vi "Print Features Report.vi"(6 "Local Data in":T2, 7 "UI References":T1, 8 "error in (no error)":errorcluster) -> (0 "error out":errorcluster)   [LabVIEW 2024]
uses:
  Controls/Print Command.ctl
  Controls/Language Vision Text Cluster.ctl
  Controls/RVHR - Reporting Settings.ctl
  Controls/RVHR - Local Data.ctl
  Controls/Test Cluster.ctl
  Controls/Excluded Information.ctl
  Controls/Language.ctl
  Controls/Device_Type.ctl
  <vilib>/Utility/miscctls.llb/LVRectTypeDef.ctl
  <vilib>/Utility/miscctls.llb/LVBoundsTypeDef.ctl
  Controls/RVHR - UI Refs.ctl
  <vilib>/drjdpowell/SQLite Library/SQL Connection/Open (path).vi
  <vilib>/drjdpowell/SQLite Library/SQL Connection/Open (string).vi
  <vilib>/AdvancedString/Path To Command Line String.vi
  <vilib>/drjdpowell/SQLite Library/SQL Connection/Execute SQL.vi
  <vilib>/drjdpowell/SQLite Library/SQL Connection/Connection.lvclass
  <vilib>/Exaprom PDF/Controls/Image Controls/Image aligment.ctl
  <vilib>/Exaprom PDF/Controls/Image Controls/Image alignment and position.ctl
  <vilib>/Exaprom PDF/Controls/Image Controls/Image border.ctl
  <vilib>/Exaprom PDF/Controls/Initialization Controls/At the opening.ctl
  <vilib>/Exaprom PDF/Controls/Page Controls/Page margins.ctl
  <vilib>/Exaprom PDF/Controls/Page Controls/Page Layout Custom.ctl
  <vilib>/Exaprom PDF/Controls/Page Controls/Page Orientation.ctl
  <vilib>/Exaprom PDF/Controls/Page Controls/Page size.ctl
  <vilib>/Exaprom PDF/Controls/Page Controls/Page setup.ctl
  <vilib>/Exaprom PDF/Controls/Initialization Controls/PDF Details.ctl
  <vilib>/Exaprom PDF/Controls/Text Controls/Unicode/Type and run direction.ctl
  <vilib>/Exaprom PDF/Controls/Font Controls/Type and encoding.ctl
  <vilib>/Exaprom PDF/Controls/Font Controls/Font color.ctl
  <vilib>/Exaprom PDF/Controls/Font Controls/Font size.ctl
  <vilib>/Exaprom PDF/Controls/Font Controls/Font complete cluster.ctl
  <vilib>/Exaprom PDF/Controls/Initialization Controls/Image or Table Caption.ctl
  <vilib>/Exaprom PDF/Controls/Initialization Controls/Captions.ctl
  <vilib>/Exaprom PDF/Controls/Text Controls/Line spacing.ctl
  <vilib>/Exaprom PDF/Controls/Text Controls/Texte alignement.ctl
  <vilib>/Exaprom PDF/Controls/Initialization Controls/Defaut Paragraphe and Line Spacing.ctl
  <vilib>/Exaprom PDF/Controls/Initialization Controls/File Permission Parameters.ctl
  <vilib>/drjdpowell/SQLite Library/SQLite.lvlib
panel:
  out "Column Names 2":string[](array[string])
  out "Feature Table":string[][](array[string])
  out "Local Data out":T2
  in  "Settings":T9
  in  "Language Config Cluster":T10={"Home"="Home", "Test Setup"="Setup", "Run Test"="Test", "Configure"="Config", "Hardware Viewer"="Viewer", "Review Test"="Review", "Report"="Home", "Exit"="Exit", "Device Connected?"="Device Connected?", "Test in Progress?"="Test in Progress?", "Simulate?"="Simulate?", "Device Type 1"="Corrugation Analysis Trolley", "Device Type 2"="Bi-Corrugation Analysis Trolley", "Device Type 3"="Bi-Corrugation Analysis Trolley", "Device Type 4"="Bi-Corrugation Analysis Trolley", "Device Type 5"="Bi-Corrugation Analysis Trolley", "Device Type 6"="Bi-Corrugation Analysis Trolley", "Device Type 7"="Bi-Corrugation Analysis Trolley", "Software Version"="Version", "Support"="Software by RailMeasurement Limited - Cambridge - UK - support@railmeasurement.com", "Operator"="Operator:", "Test Description"="Description:", "Line"="Description:", "Test Folder Path"="Folder Path:", "Test Folder Path RCA"="Folder Path:", "Start Position"="Start Position:", "Sensor Position"="Sensor Position:", "Sensor A Position"="Sensor A Position:", "Sensor B Position"="Sensor B Position:", "Visible Chart Distance"="Sensor B Position:", "Rail Side"="Rail Side:", "Rail A Side"="Rail A Side:", "Distance Direction"="Distance Direction:", "Start"="Start:", "Distance Travelled"="Distance Travelled:", "Current Position"="Current Position:", "Stop Test"="Stop", "Pause Test"="Save", "Displacement"="Displacement", "Position"="Position", "Sensor Calibration"="Sensor Calibration:", "Sensor A Calibration"="Sensor A Calibration:", "Sensor B Calibration"="Sensor B Calibration:", "Encoder Spacing"="Encoder Spacing:", "Sampling Distance"="Sampling Distance:", "Tacho Pulses/Rev"="Sensor Calibration:", "Wheel Diameter"="Sensor A Calibration:", "Sampling Distances"=["1mm", "2mm"], "Distance Unit"="Distance in:", "Distance Units"=["Kilometres", "miles & chains", "metres", "stations", "miles"], "Swap Direction"="Swap Direction at Run End?", "Language"="Language", "Device Resolution"="Save", "Device Resolutions"=["Kilometres", "miles & chains", "metres", "stations", "miles"], "Detect Change in Direction"="Save", "Save Config"="Save", "Encoder Data"="Encoder Data", "Sensor Data"="Sensor Data", "Sensor A Data"="Sensor A Data", "Sensor B Data"="Sensor B Data", "Voltage"="Voltage", "Time (m:s)"="Time (m:s)", "Unit mm/s/V"="(mm/s)/V", "Unit mm"="mm", "Unit km"="km", "Unit m"="m", "Start Test Message"="m", "Stop Test Message"="km", "Exit Message"="mm", "File Exists Message"="mm", "File Path Invalid Message"="mm", "Combine Error"="mm", "Combine Success"="mm", "Roller Comp Error"="mm", "Test Folder Path (Live)"="mm", "Folder Error"="Sensor B Position:", "Enc Count"="Setup", "Run Start"="mm", "Run End"="mm", "Date"="mm", "Train"="Sensor B Position:", "Location"="Setup", "Notes"="mm", "Heading_1"="mm", "Heading_2"="mm", "Left Rail"="Sensor B Position:", "Right Rail"="Setup", "Left Exclusions"="mm", "Right Exclusions"="mm", "Settings"="mm", "Wavelength Ranges"="Sensor B Position:", "Y-Axis Limits"="Setup", "Exc Limits"="Sensor B Position:", "Other Settings"="Setup", "Distance/Page"="mm", "Distance/Pages"=["Kilometres", "miles & chains", "metres", "stations", "miles"], "Gridlines"="mm", "Report Tolerance"="mm", "Manual Cut"="Sensor B Position:", "Plot Colour"="Distance in:", "Plot Colours"=["Kilometres", "miles & chains", "metres", "stations", "miles"], "EN Standard"="mm", "RiL Standard"="mm", "Custom Standard"="mm", "Resolution"="Distance in:", "Resolutions"=["Kilometres", "miles & chains", "metres", "stations", "miles"], "Exceedence Header"="mm", "Distance (km)"="mm", "Left (%)"="mm", "Right (%)"="Distance in:", "Page"="Distance in:", "Align"="mm", "Main"="mm", "Comparison"="Distance in:", "Offset"="Distance in:", "From"="Distance in:", "To"="Distance in:", "Of"="Distance in:", "File"="mm", "Load New"="mm", "Load Comparison"="Distance in:", "Discard Comparison"="Distance in:", "Print Current Page"="Distance in:", "Print All Pages"="Distance in:", "Print Exceedence Report"="Distance in:", "Plot Main"="Distance in:", "No Comparison Data to Align"="Distance in:", "Run Load Error"="Distance in:", "Report Load Error"="Distance in:", "Cut"="Distance in:", "Remove"="Distance in:", "Config Settings Unsaved"="Distance in:", "Acquisition Paused"="Distance in:", "Please Select One Option Below"="Distance in:", "RCA is Now Stationary"="Distance in:", "Reporting Setting"="Distance in:", "Main Abbreviated"="Distance in:", "Comparison Abbreviated"="Distance in:", "Exceedence Abbreviated"="Distance in:", "Align Comparison"="Distance in:", "Rail Corrugation Analyser Reporting"="Distance in:", "Show Exc. % in Graph"="Distance in:", "Evaluate Sections <100m"="Distance in:", "Evaluate Sections <0.062mile"="Distance in:", "Section Too Short for Evaluation"="Distance in:", "Language Change Prompt"="Distance in:", "Show All"="Distance in:", "Sections_km"="Distance in:", "Sections_mi"="Distance in:", "Vision"="Distance in:", "Vision Report"="Distance in:", "Vision Display"="Distance in:", "Vision Displays"=["Kilometres", "miles & chains", "metres", "stations", "miles"], "Save Images"="Distance in:", "Image Frequency"="Distance in:", "Section"="Distance in:", "Brightness"="Distance in:", "Contrast"="Distance in:", "Shadow"="Distance in:", "Sharpened"="Distance in:", "Apply to all Images"="Distance in:", "Reset"="Distance in:", "Are you sure"="Distance in:", "Image Processing"="Distance in:", "Save Video"="Distance in:", "Image Offset"="Distance in:", "Camera Mode"="Distance in:", "Camera Modes"=["Kilometres", "miles & chains", "metres", "stations", "miles"], "Copy Page"="Distance in:", "Copy Graphs"="Distance in:", "Camera Mode Change Prompt"="Distance in:", "Camera_1 Missing"="Distance in:", "Camera_2 Missing"="Distance in:", "Cameras Missing"="Distance in:", "Camera Setup"="Distance in:", "Camera_1 Connection Error"="Distance in:", "Camera_2 Connection Error"="Distance in:", "Cameras Connection Error"="Distance in:", "No GPS"="Distance in:", "No Signal"="Distance in:", "Camera_1 Connected"="Distance in:", "Camera_1 Not Connected"="Distance in:", "Camera_2 Connected"="Distance in:", "Camera_2 Not Connected"="Distance in:", "Start Position at 0m?"="Distance in:", "Continue"="Distance in:", "New Test, Same Direction"="Distance in:", "New Test, Opposite Direction"="Distance in:", "Stop and Save"="Distance in:", "Live Corrug Estimate"="Distance in:", "Wavelength Corrug"="Distance in:", "Distance Corrug "="Distance in:", "Update Corrug"="Distance in:", "Company"="Distance in:", "Ref Profile "="Distance in:", "Company_Report"="Distance in:", "Ref Profile_Report"="Distance in:", "Heading_1_RVHR"="Distance in:", "Heading_2_RVHR"="Distance in:", "Remove Feature"="Distance in:", "Feature Type"="Sampling Distance:", "Feature Types"=["1mm", "2mm"], "AI Not Ready"="Sampling Distance:"}
  in  "Command":T11
  in  "Main VI Path":path
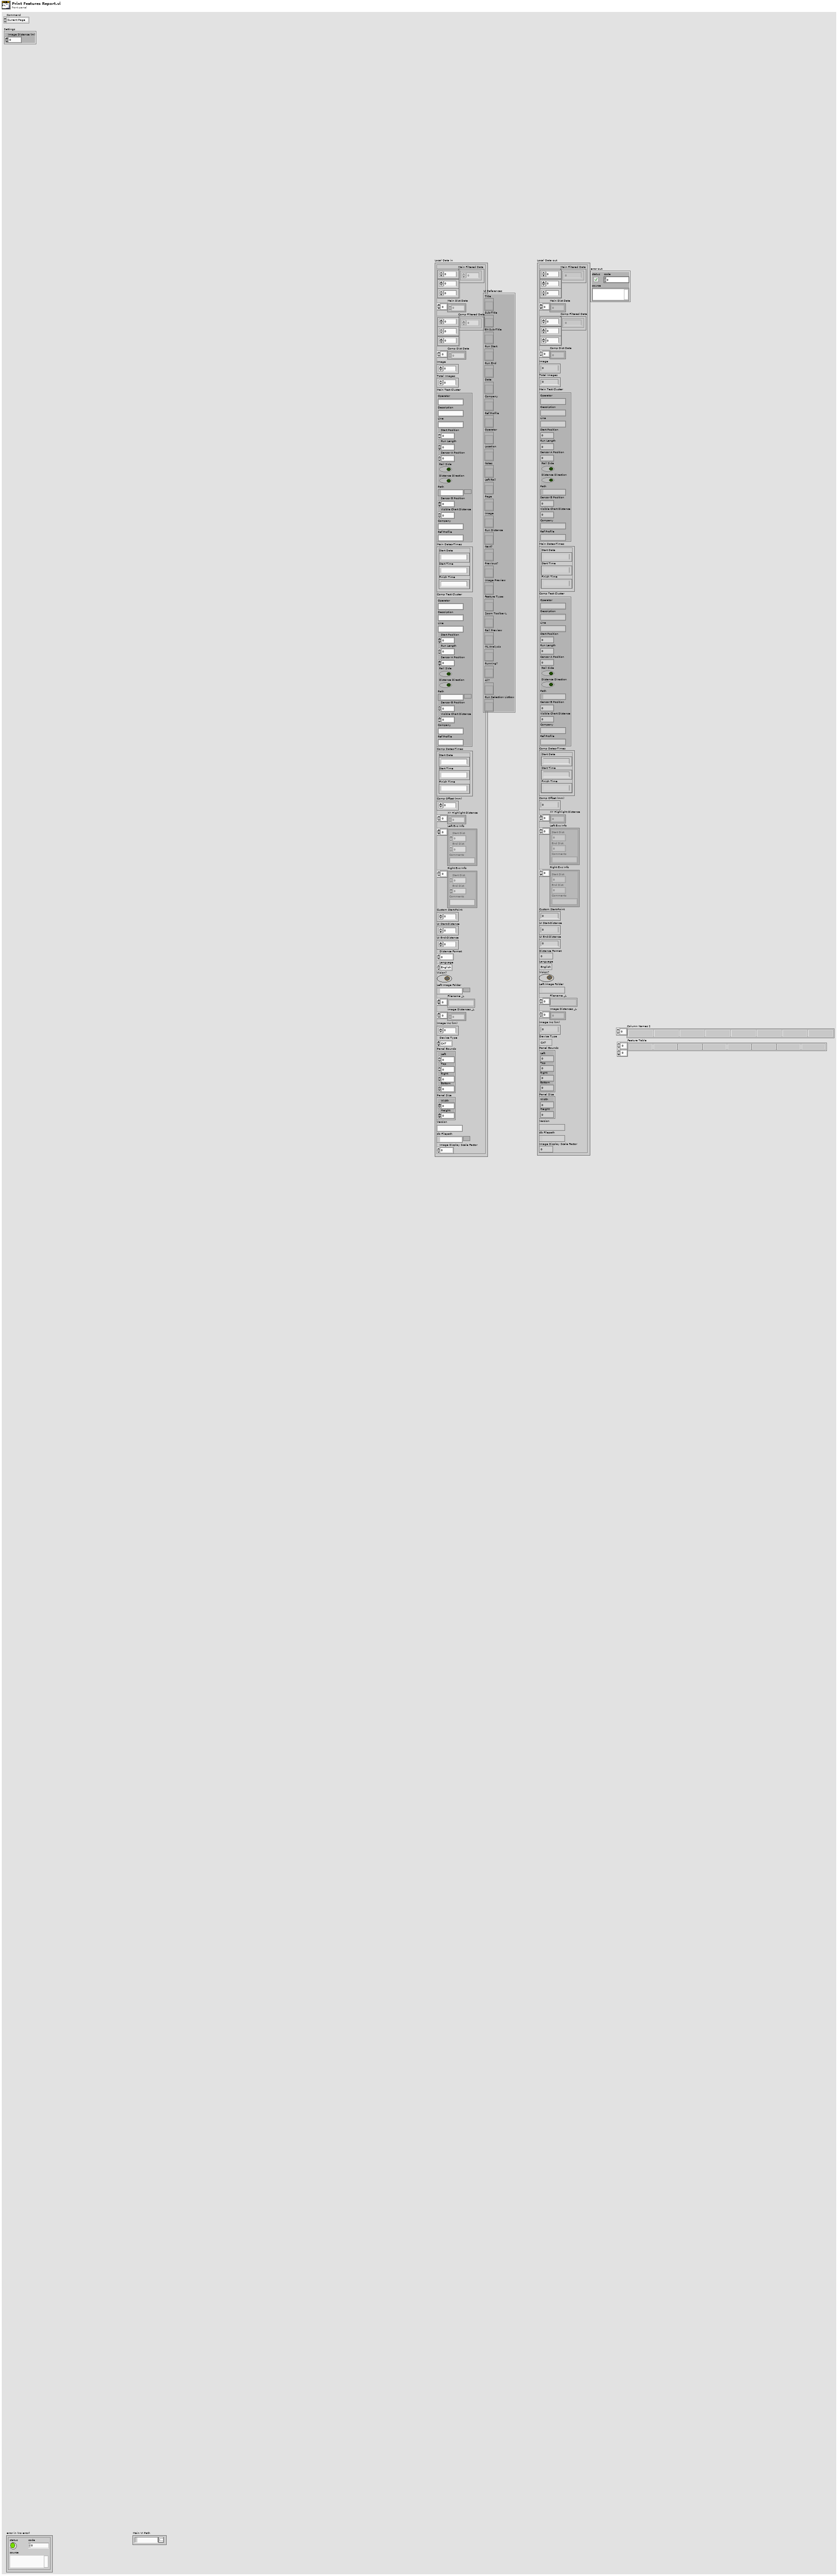
[diagram p1: front panel]
types:
  T1 = typedef "RVHR - UI Refs.ctl" = cluster{"Title":refnum<vi>, "Sub-Title":refnum<vi>, "EN Sub-Title":refnum<vi>, "Run Start":refnum<vi>, "Run End":refnum<vi>, "Date":refnum<vi>, "Company":refnum<vi>, "Ref Profile":refnum<vi>, "Operator":refnum<vi>, "Location":refnum<vi>, "Notes":refnum<vi>, "Left Rail":refnum<vi>, "Page":refnum<vi>, "Image":refnum<vi>, "Run Distance":refnum<vi>, "Next?":refnum<vi>, "Previous?":refnum<vi>, "Image Preview":refnum<vi>, "Feature Type:":refnum<vi>, "Zoom Toolbar L":refnum<vi>, "Rail Preview":refnum<vi>, "ML Analysis":refnum<vi>, "Running?":refnum<vi>, "All?":refnum<vi>, "Run Selection Listbox":refnum<vi>}
  T2 = typedef "RVHR - Local Data.ctl" = cluster{"Main Filtered Data":dbl[][][], "Main Dist Data":dbl[], "Comp Filtered Data":dbl[][][], "Comp Dist Data":dbl[], "Image":u16, "Total Images":u16, "Main Test Cluster":T3, "Main Dates-Times":cluster{"Start Date":string, "Start Time":string, "Finish Time":string}, "Comp Test Cluster":T3, "Comp Dates-Times":cluster{"Start Date":string, "Start Time":string, "Finish Time":string}, "Comp Offset (mm)":i64, "XY Highlight Distance":dbl[], "Left Exc Info":T4[], "Right Exc Info":T4[], "Custom Start-Point":dbl, "UI Start-Distance":dbl, "UI End-Distance":dbl, "Distance Format":u8, "Language":T5, "Vision?":bool, "Left Image Folder":path, "Filename _L":string[], "Image Distances _L":dbl[], "Image Inc (km)":dbl, "Device Type":T6, "Panel Bounds":T7, "Panel Size":T8, "Version":string, "db Filepath":path, "Image Display Scale Factor":dbl}
  T3 = typedef "Test Cluster.ctl" = cluster{"Operator":string, "Description":string, "Line":string, "Start Position":dbl, "Run Length":dbl, "Sensor A Position":dbl, "Rail Side":bool, "Distance Direction":bool, "Path":path, "Sensor B Position":dbl, "Visible Chart Distance":dbl, "Company":string, "Ref Profile":string}
  T4 = typedef "Excluded Information.ctl" = cluster{"Start Dist":dbl, "End Dist":dbl, "Comments":string}
  T5 = typedef "Language.ctl" = enum16{"English", "Chinese", "German"}
  T6 = typedef "Device_Type.ctl" = enum16{"CAT", "Bi-CAT", "YRCA", "RCA", "RV-HR", "TV-HR"}
  T7 = typedef "LVRectTypeDef.ctl" = cluster{"Left":i16, "Top":i16, "Right":i16, "Bottom":i16}
  T8 = typedef "LVBoundsTypeDef.ctl" = cluster{"Width":u32, "Height":u32}
  T9 = typedef "RVHR - Reporting Settings.ctl" = cluster{"Image Distance (m)":dbl}
  T10 = typedef "Language Vision Text Cluster.ctl" = cluster{"Home":string, "Test Setup":string, "Run Test":string, "Configure":string, "Hardware Viewer":string, "Review Test":string, "Report":string, "Exit":string, "Device Connected?":string, "Test in Progress?":string, "Simulate?":string, "Device Type 1":string, "Device Type 2":string, "Device Type 3":string, "Device Type 4":string, "Device Type 5":string, "Device Type 6":string, "Device Type 7":string, "Software Version":string, "Support":string, "Operator":string, "Test Description":string, "Line":string, "Test Folder Path":string, "Test Folder Path RCA":string, "Start Position":string, "Sensor Position":string, "Sensor A Position":string, "Sensor B Position":string, "Visible Chart Distance":string, "Rail Side":string, "Rail A Side":string, "Distance Direction":string, "Start":string, "Distance Travelled":string, "Current Position":string, "Stop Test":string, "Pause Test":string, "Displacement":string, "Position":string, "Sensor Calibration":string, "Sensor A Calibration":string, "Sensor B Calibration":string, "Encoder Spacing":string, "Sampling Distance":string, "Tacho Pulses/Rev":string, "Wheel Diameter":string, "Sampling Distances":string[], "Distance Unit":string, "Distance Units":string[], "Swap Direction":string, "Language":string, "Device Resolution":string, "Device Resolutions":string[], "Detect Change in Direction":string, "Save Config":string, "Encoder Data":string, "Sensor Data":string, "Sensor A Data":string, "Sensor B Data":string, "Voltage":string, "Time (m:s)":string, "Unit mm/s/V":string, "Unit mm":string, "Unit km":string, "Unit m":string, "Start Test Message":string, "Stop Test Message":string, "Exit Message":string, "File Exists Message":string, "File Path Invalid Message":string, "Combine Error":string, "Combine Success":string, "Roller Comp Error":string, "Test Folder Path (Live)":string, "Folder Error":string, "Enc Count":string, "Run Start":string, "Run End":string, "Date":string, "Train":string, "Location":string, "Notes":string, "Heading_1":string, "Heading_2":string, "Left Rail":string, "Right Rail":string, "Left Exclusions":string, "Right Exclusions":string, "Settings":string, "Wavelength Ranges":string, "Y-Axis Limits":string, "Exc Limits":string, "Other Settings":string, "Distance/Page":string, "Distance/Pages":string[], "Gridlines":string, "Report Tolerance":string, "Manual Cut":string, "Plot Colour":string, "Plot Colours":string[], "EN Standard":string, "RiL Standard":string, "Custom Standard":string, "Resolution":string, "Resolutions":string[], "Exceedence Header":string, "Distance (km)":string, "Left (%)":string, "Right (%)":string, "Page":string, "Align":string, "Main":string, "Comparison":string, "Offset":string, "From":string, "To":string, "Of":string, "File":string, "Load New":string, "Load Comparison":string, "Discard Comparison":string, "Print Current Page":string, "Print All Pages":string, "Print Exceedence Report":string, "Plot Main":string, "No Comparison Data to Align":string, "Run Load Error":string, "Report Load Error":string, "Cut":string, "Remove":string, "Config Settings Unsaved":string, "Acquisition Paused":string, "Please Select One Option Below":string, "RCA is Now Stationary":string, "Reporting Setting":string, "Main Abbreviated":string, "Comparison Abbreviated":string, "Exceedence Abbreviated":string, "Align Comparison":string, "Rail Corrugation Analyser Reporting":string, "Show Exc. % in Graph":string, "Evaluate Sections <100m":string, "Evaluate Sections <0.062mile":string, "Section Too Short for Evaluation":string, "Language Change Prompt":string, "Show All":string, "Sections_km":string, "Sections_mi":string, "Vision":string, "Vision Report":string, "Vision Display":string, "Vision Displays":string[], "Save Images":string, "Image Frequency":string, "Section":string, "Brightness":string, "Contrast":string, "Shadow":string, "Sharpened":string, "Apply to all Images":string, "Reset":string, "Are you sure":string, "Image Processing":string, "Save Video":string, "Image Offset":string, "Camera Mode":string, "Camera Modes":string[], "Copy Page":string, "Copy Graphs":string, "Camera Mode Change Prompt":string, "Camera_1 Missing":string, "Camera_2 Missing":string, "Cameras Missing":string, "Camera Setup":string, "Camera_1 Connection Error":string, "Camera_2 Connection Error":string, "Cameras Connection Error":string, "No GPS":string, "No Signal":string, "Camera_1 Connected":string, "Camera_1 Not Connected":string, "Camera_2 Connected":string, "Camera_2 Not Connected":string, "Start Position at 0m?":string, "Continue":string, "New Test, Same Direction":string, "New Test, Opposite Direction":string, "Stop and Save":string, "Live Corrug Estimate":string, "Wavelength Corrug":string, "Distance Corrug ":string, "Update Corrug":string, "Company":string, "Ref Profile ":string, "Company_Report":string, "Ref Profile_Report":string, "Heading_1_RVHR":string, "Heading_2_RVHR":string, "Remove Feature":string, "Feature Type":string, "Feature Types":string[], "AI Not Ready":string}
  T11 = typedef "Print Command.ctl" = enum16{"Current Page", "Full Report"}
  T12 = typedef "File Permission Parameters.ctl" = cluster{"User Password":string, "Owner Password":string, "Printing":enum16{"Allow Printing", "Allow Degraded Printing", "Don't Allow Printing"}, "Allow Modify Contents":bool, "Allow Copy":bool, "Allow Modify Annotations":bool, "Allow Fill In ":bool, "Allow Screen Readers":bool, "Allow Assembly":bool}
  T13 = typedef "Captions.ctl" = cluster{"Figure":T14, "Table":T14, "Font":T15}
  T14 = typedef "Image or Table Caption.ctl" = cluster{"Caption":string, "Separator":string, "Position":enum16{"Above", "Below"}}
  T15 = typedef "Font complete cluster.ctl" = cluster{"Name":string, "Size":T16, "Color":T17, "Style":cluster{"Bold":bool, "Italic":bool, "Underline":bool, "Strikeout":bool}, "Type":T18}
  T16 = typedef "Font size.ctl" = sgl
  T17 = typedef "Font color.ctl" = u32
  T18 = typedef "Type and encoding.ctl" = cluster{"Type&direction":T19, "Embedded":bool, "Encoding":string}
  T19 = typedef "Type and run direction.ctl" = enum16{"Select", "ASCII", "UTF-16", "UTF-16 (default)", "UTF-16 (LTR)", "UTF-16 (RTL)"}
  T20 = typedef "Defaut Paragraphe and Line Spacing.ctl" = cluster{" Aligment":T21, "Line spacing":T22}
  T21 = typedef "Texte alignement.ctl" = enum16{"Select", "CENTER", "JUSTIFY", "LEFT", "RIGHT"}
  T22 = typedef "Line spacing.ctl" = enum16{"Select", "1.0", "1.5", "2.0"}
  T23 = typedef "PDF Details.ctl" = cluster{"Title":string, "Author":string, "Subject":string, "Keywords":string, "Creator":string}
  T24 = typedef "Page setup.ctl" = cluster{"Page Size":T25, "Orientation":T26, "Custom Size":T27, "Margins":T28}
  T25 = typedef "Page size.ctl" = i32
  T26 = typedef "Page Orientation.ctl" = enum16{"Portrait", "Landscape"}
  T27 = typedef "Page Layout Custom.ctl" = cluster{"Width":sgl, "Height":sgl}
  T28 = typedef "Page margins.ctl" = cluster{"Left":sgl, "Right":sgl, "Top":sgl, "Bottom":sgl}
  T29 = typedef "At the opening.ctl" = cluster{"Page":u16, "Show Bookmarks":bool}
  T30 = typedef "Image alignment and position.ctl" = cluster{"Alignment":T31, "X ":sgl, "Y":sgl, "Indentation":sgl}
  T31 = typedef "Image aligment.ctl" = enum16{"Absolute (X,Y)", "Left", "Center", "Right", "Left (textwrap)", "Right (textwrap)"}
  T32 = typedef "Image border.ctl" = cluster{"Show?":bool, "Thickness (point)":sgl, "Color":u32}
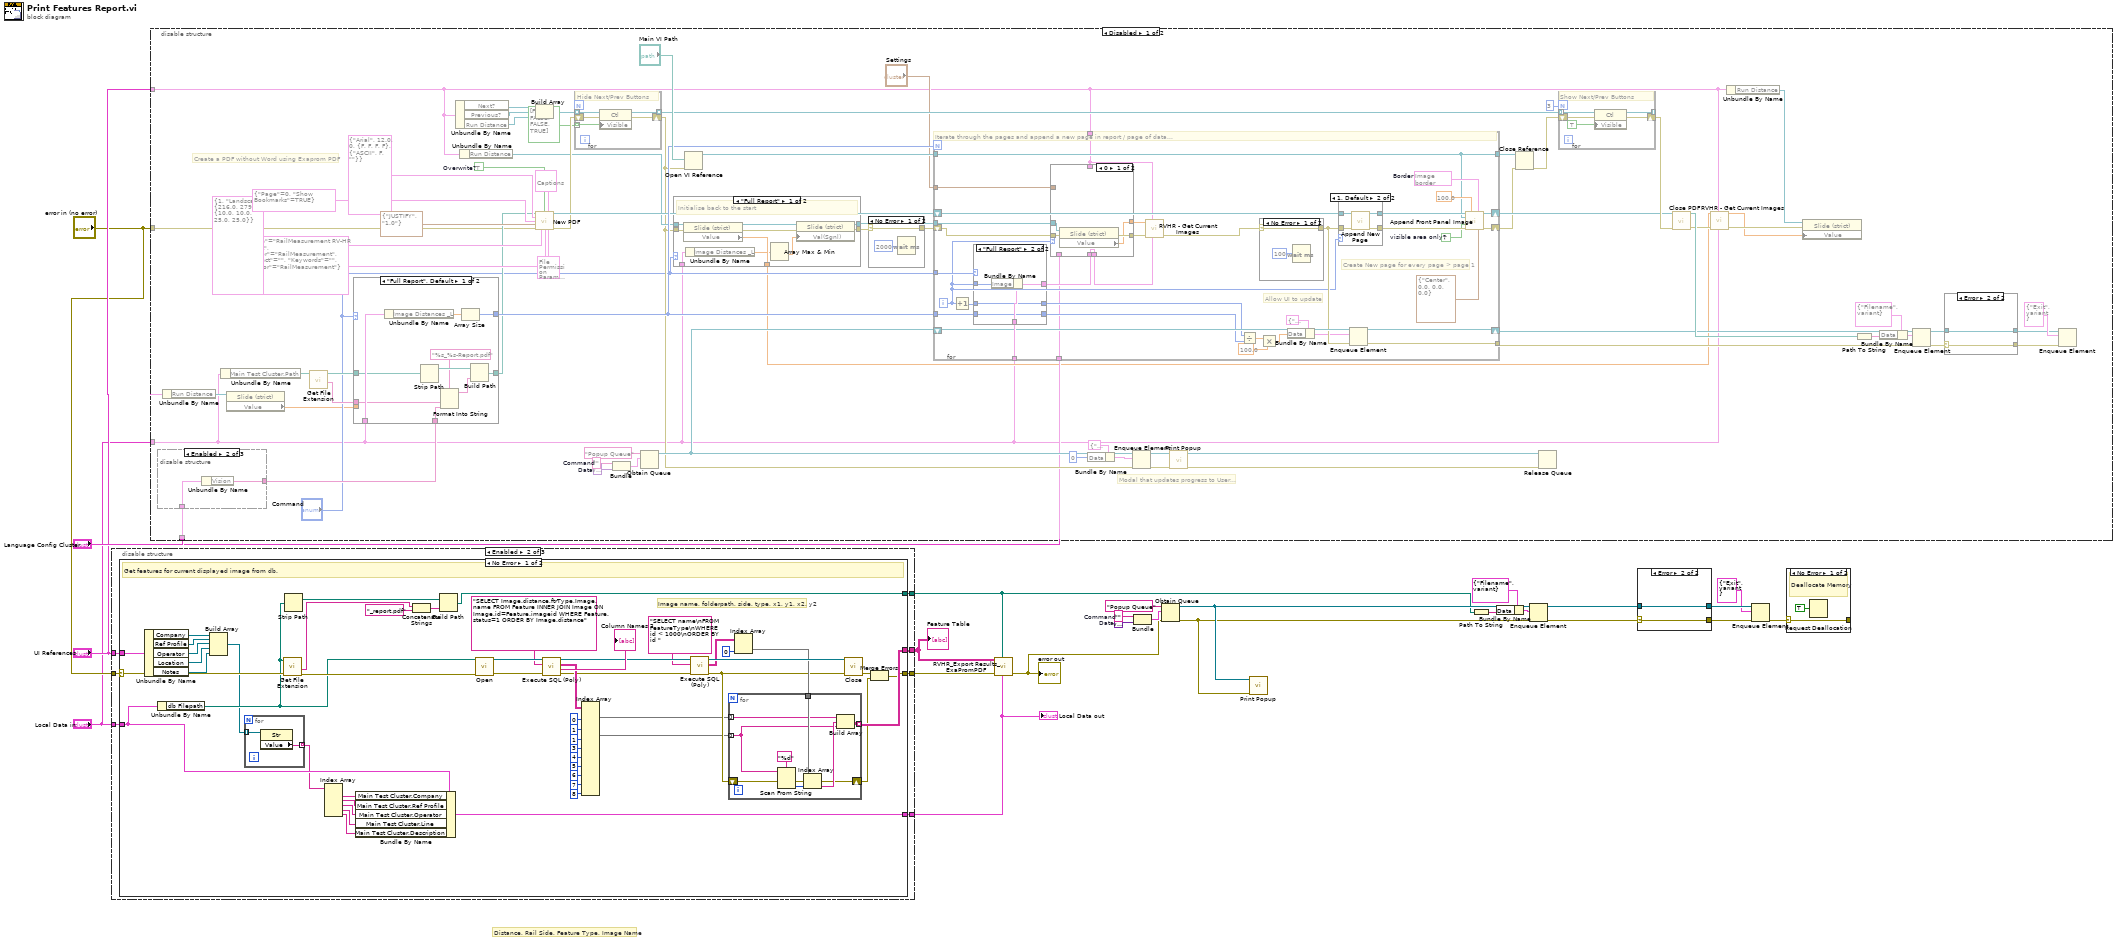
[diagram p0: block diagram]
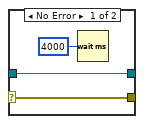
[diagram p3: hidden frame]
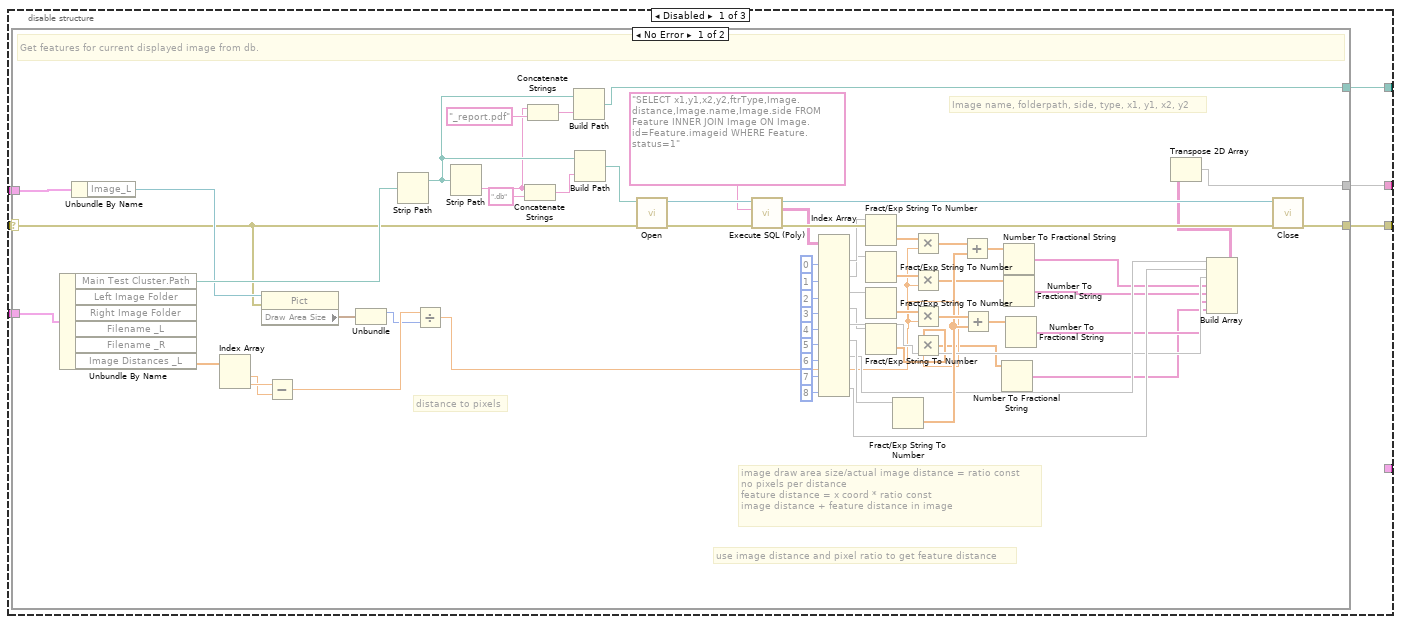
[diagram p4: hidden frame]
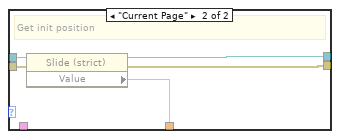
[diagram p8: hidden frame]
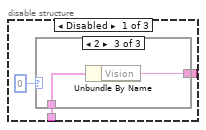
[diagram p10: hidden frame]
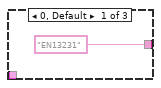
[diagram p11: hidden frame]
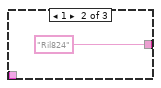
[diagram p12: hidden frame]
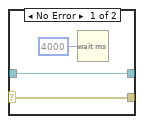
[diagram p14: hidden frame]
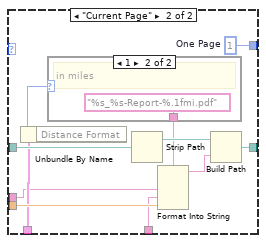
[diagram p15: hidden frame]
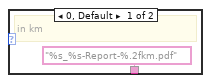
[diagram p16: hidden frame]
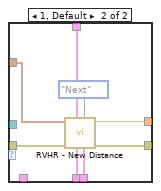
[diagram p17: hidden frame]
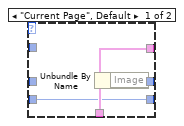
[diagram p19: hidden frame]
diagram:
  w18 = variant  # Data
  w17 = ""  # Command
  # "Distance, Rail Side, Feature Type, Image Name"
  n1 = disable-structure shown="Enabled" {
    disable-tunnel: "Local Data in" -> [w30 w100 _]
    disable-tunnel: "UI References" -> [w29 w99 _]
    disable-tunnel: "error in (no error)" -> [w28 w98 _]
    disable-tunnel: [w27 w97 _] -> w21
    disable-tunnel: [w26 w96 _] -> w5
    disable-tunnel: [w25 w95 _] -> w20
    disable-tunnel: [_ w94 _] -> w1
    frame Disabled {
      n2 = case shown="No Error" w28 {
        selector: w28 -> [w64 w93]
        tunnel: w30 -> [w91 _]
        tunnel: [w92 w93] -> w25
        tunnel: w29 -> [w90 _]
        tunnel: [w89 _] -> w27
        tunnel: [w32 _] -> w26
        frame No Error {
          # "Image name, folderpath, side, type, x1, y1, x2, y2"
          # "image draw area size/actual image distance = ratio const\nno pixels per distance\nfeature distance = x coord * ratio const\nimage distance + feature distance in image"
          # "use image distance and pixel ratio to get feature distance"
          # "distance to pixels"
          # "Get features for current displayed image from db."
          n3 = Unbundle By Name(w91) -> ("Main Test Cluster.Path"=w88:path, "Image Distances _L"=w79:dbl[])  [unwired: 4 out]
          n4 = Unbundle By Name(w90) -> ("Image_L"=w65:refnum<vi>)
          n5 = Index Array(array=w79) -> (element #1=w77:dbl, element #2=w78:dbl)  [unwired: 2 in]
          n6 = property class="Pict"(reference=w65, error in=w64) -> ("Draw Area Size"=w80:T8)  [unwired: 2 out]
          n7 = Subtract(x=w78, y=w77) -> (x-y=w59:dbl)
          n8 = Unbundle(w80) -> ("Width"=w58:u32)  [unwired: 1 out]
          n9 = Strip Path(path=w88) -> (stripped path=w34:path)  [unwired: 1 out]
          n10 = Divide(x=w59, y=w58) -> (x/y=w39:dbl)
          n11 = Strip Path(path=w34) -> (name=w33:string)  [unwired: 1 out]
          n12 = Concatenate Strings(w33, ".db" ("string")) -> (w87:string)
          n13 = Concatenate Strings(w33, "_report.pdf") -> (w36:string)
          n14 = Build Path(base path=w34, name or relative path=w36) -> (appended path=w32:path)
          n15 = Build Path(base path=w34, name or relative path=w87) -> (appended path=w85:path)
          n16 = call-poly <vilib>:"Open.vi"("error in (no error)"=w64, "db file"=w85) -> ("error out"=w84:errorcluster, "SQLite Connection"=w83:refnum<class "Connection.lvclass">)  [unwired: 8 in]
          n17 = call-poly <vilib>:"Execute SQL (Poly).vi"("error in (no error)"=w84, "SQL"="SELECT x1,y1,x2,y2,ftrType,Image.distance,Image.name,Image.side FROM Feature INNER JOIN Image ON Image.id=Feature.imageid WHERE Feature.status=1" ("format string"), "SQLite Connection in"=w83) -> ("error out"=w81:errorcluster, "Column Names"=w31:string[], "Result Set"=w76:string[][], "SQLite Connection"=w82:refnum<class "Connection.lvclass">)  [unwired: 5 in]
          n18 = Index Array(array=w76, index (col) #1=0 ("disabled index (col)"), index (col) #2=1 ("index (col)"), index (col) #3=2 ("index (col)"), index (col) #4=3 ("index (col)"), index (col) #5=4 ("index (col)"), index (col) #6=5 ("index (col)"), index (col) #7=6 ("index (col)"), index (col) #8=7 ("index (col)"), index (col) #9=8 ("index (col)")) -> (element #1=w62:string[], element #2=w45:string[], element #3=w60:string[], element #4=w41:string[], element #5=w48:string[], element #6=w75:string[], element #7=w50:string[], element #9=w49:string[])  [unwired: 9 in, 1 out]
          n19 = Fract/Exp String To Number(string=w62) -> (number=w63:dbl[])  [unwired: 3 in, 1 out]
          n20 = Fract/Exp String To Number(string=w45) -> (number=w44:dbl[])  [unwired: 3 in, 1 out]
          n21 = Fract/Exp String To Number(string=w60) -> (number=w61:dbl[])  [unwired: 3 in, 1 out]
          n22 = Fract/Exp String To Number(string=w41) -> (number=w40:dbl[])  [unwired: 3 in, 1 out]
          n23 = Fract/Exp String To Number(string=w75) -> (number=w55:dbl[])  [unwired: 3 in, 1 out]
          n24 = Multiply(x=w63, y=w39) -> (x*y=w57:dbl[])
          n25 = Multiply(x=w44, y=w39) -> (x*y=w43:dbl[])
          n26 = Multiply(x=w61, y=w39) -> (x*y=w56:dbl[])
          n27 = Multiply(x=w40, y=w39) -> (x*y=w38:dbl[])
          n28 = Add(x=w57, y=w55) -> (x+y=w74:dbl[])
          n29 = Add(x=w56, y=w55) -> (x+y=w54:dbl[])
          n30 = Number To Fractional String(number=w38) -> (F-format string=w37:string[])  [unwired: 3 in]
          n31 = Number To Fractional String(number=w74) -> (F-format string=w47:string[])  [unwired: 3 in]
          n32 = Number To Fractional String(number=w43) -> (F-format string=w42:string[])  [unwired: 3 in]
          n33 = Number To Fractional String(number=w54) -> (F-format string=w46:string[])  [unwired: 3 in]
          n34 = Build Array(w50, w49, w48, w47, w42, w46, w37) -> (w67:string[][])
          n35 = Transpose 2D Array(2D array=w67) -> (transposed array=w89:string[][])
          n36 = call-dynamic "Close.vi"("error in (no error)"=w81, "SQLite Connection in"=w82) -> ("error out"=w92:errorcluster)  [unwired: 9 in]
        }
        frame Error {
        }
      }
    }
    frame Enabled {
      n37 = case shown="No Error" w98 {
        selector: w98 -> [w119 w164]
        tunnel: w100 -> [w108 w163]
        tunnel: [w121 w164] -> w95
        tunnel: w99 -> [w150 _]
        tunnel: [w122 _] -> w97
        tunnel: [w135 _] -> w96
        tunnel: [w101 w163] -> w94
        frame No Error {
          # "Image name, folderpath, side, type, x1, y1, x2, y2"
          # "Get features for current displayed image from db."
          n38 = Unbundle By Name(w150) -> ("Company"=w114:refnum<vi>, "Ref Profile"=w113:refnum<vi>, "Operator"=w112:refnum<vi>, "Location"=w111:refnum<vi>, "Notes"=w110:refnum<vi>)
          n39 = Unbundle By Name(w108) -> ("db Filepath"=w116:path)
          n40 = Build Array(w114, w113, w112, w111, w110) -> (w109:refnum<vi>[])
          n41 = for {
            tunnel: w109 -> [w153] mode=indexing
            tunnel: [w152] -> w107 mode=indexing
            n42 = property class="Str"(reference=w153) -> ("Value"=w152:string)  [unwired: 1 in, 2 out]
          }
          n43 = call <vilib>:"Get File Extension.vi"("error in (no error)"=w119, "file"=w116) -> ("error out"=w118:errorcluster, "filename without extension"=w117:string)  [unwired: 5 in, 3 out]
          n44 = Strip Path(path=w116) -> (stripped path=w115:path)  [unwired: 1 out]
          n45 = Index Array(array=w107) -> (element #1=w106:string, element #2=w105:string, element #3=w104:string, element #4=w103:string, element #5=w102:string)  [unwired: 5 in]
          n46 = Bundle By Name(cluster=w108, "Main Test Cluster.Company"=w106, "Main Test Cluster.Ref Profile"=w105, "Main Test Cluster.Operator"=w104, "Main Test Cluster.Line"=w103, "Main Test Cluster.Description"=w102) -> (w101:T2)
          n47 = Concatenate Strings(w117, "_report.pdf") -> (w137:string)
          n48 = Build Path(base path=w115, name or relative path=w137) -> (appended path=w135:path)
          n49 = call-poly <vilib>:"Open.vi"("error in (no error)"=w118, "db file"=w116) -> ("error out"=w149:errorcluster, "SQLite Connection"=w148:refnum<class "Connection.lvclass">)  [unwired: 8 in]
          n50 = call-poly <vilib>:"Execute SQL (Poly).vi"("error in (no error)"=w149, "SQL"="SELECT Image.distance,ftrType,Image.name FROM Feature INNER JOIN Image ON Image.id=Feature.imageid WHERE Feature.status=1 ORDER BY Image.distance" ("format string"), "SQLite Connection in"=w148) -> ("error out"=w132:errorcluster, "Column Names"=→"Column Names 2":string[], "Result Set"=w133:string[][], "SQLite Connection"=w131:refnum<class "Connection.lvclass">)  [unwired: 5 in]
          n51 = Index Array(array=w133, index (col) #1=0 ("disabled index (col)"), index (col) #2=1 ("index (col)"), index (col) #3=1 ("index (col)"), index (col) #4=3 ("index (col)"), index (col) #5=4 ("index (col)"), index (col) #6=5 ("index (col)"), index (col) #7=6 ("index (col)"), index (col) #8=7 ("index (col)"), index (col) #9=8 ("index (col)")) -> (element #1=w124:string[], element #3=w123:string[])  [unwired: 9 in, 7 out]
          n52 = call-poly <vilib>:"Execute SQL (Poly).vi"("error in (no error)"=w132, "SQL"="SELECT name\nFROM FeatureType\nWHERE id < 1000\nORDER BY id ", "SQLite Connection in"=w131) -> ("error out"=w125:errorcluster, "Result Set"=w128:string[][], "SQLite Connection"=w130:refnum<class "Connection.lvclass">)  [unwired: 5 in, 1 out]
          n53 = Index Array(array=w128, index (col)=0 ("disabled index (col)")) -> (element=w126:string[])  [unwired: 1 in]
          n54 = for {
            tunnel: w126 -> [w159]
            shift-right: [w155] -> w120
            shift-left: w125 -> [w160]
            tunnel: w124 -> [w158] mode=indexing
            tunnel: w123 -> [w154] mode=indexing
            tunnel: [w156] -> w122 mode=indexing
            n55 = Scan From String(format string="%d", input string=w154, error in=w160) -> (error out=w155:errorcluster, output 1=w161:i32)  [unwired: 2 in, 2 out]
            n56 = Index Array(array=w159, index=w161) -> (element=w157:string)
            n57 = Build Array(w158, w157, w154) -> (w156:string[])
          }
          n58 = call-dynamic "Close.vi"("error in (no error)"=w125, "SQLite Connection in"=w130) -> ("error out"=w151:errorcluster)  [unwired: 9 in]
          n59 = Merge Errors(w151, w120) -> (w121:errorcluster)
        }
        frame Error {
        }
      }
    }
    frame Disabled {
    }
  }
  "Local Data out" <- w1
  "Feature Table" <- w21
  n60 = disable-structure shown="Disabled" {
    disable-tunnel: "Language Config Cluster" -> [w175 _]
    disable-tunnel: "Local Data in" -> [w167 _]
    disable-tunnel: "UI References" -> [w166 _]
    disable-tunnel: "error in (no error)" -> [w165 _]
    frame Disabled {
      w205 = TRUE  # Overwrite?
      w217 = variant  # Data
      w226 = ""  # Command
      # "Create a PDF without Word using Exaprom PDF"
      # "Modal that updates progress to User..."
      n61 = disable-structure shown="Enabled" {
        disable-tunnel: [w255 w261 _] -> w186
        disable-tunnel: w175 -> [w254 w260 _]
        frame Disabled {
          n62 = case shown="2" 0 ("index of element") {
            tunnel: ["EN13231" ("Creator") "Ril824" ("Creator") w259] -> w255
            tunnel: w254 -> [_ _ w258]
            frame 0, Default {
            }
            frame 1 {
            }
            frame 2 {
              n63 = Unbundle By Name(w258) -> ("Vision"=w259:string)
            }
          }
        }
        frame Enabled {
          n64 = Unbundle By Name(w260) -> ("Vision"=w261:string)
        }
        frame Disabled {
        }
      }
      n65 = Unbundle By Name(w166) -> ("Run Distance"=w185:refnum<vi>)
      n66 = Unbundle By Name(w167) -> ("Main Test Cluster.Path"=w233:path)
      n67 = property class="Slide (strict)"(reference=w185) -> ("Value"=w173:dbl)  [unwired: 1 in, 2 out]
      n68 = call <vilib>:"Get File Extension.vi"("file"=w233) -> ("filename without extension"=w218:string, "dup file"=w219:path)  [unwired: 6 in, 3 out]
      n69 = case shown="\"Full Report\", Default" "Command" {
        tunnel: [w268 w282] -> w232
        tunnel: w167 -> [w276 w280]
        tunnel: w219 -> [w274 w286]
        tunnel: [w273 w285] -> w196
        tunnel: w218 -> [w271 w278]
        tunnel: w173 -> [_ w284]
        tunnel: w186 -> [w269 w277]
        frame "Full Report", Default {
          n70 = Unbundle By Name(w276) -> ("Image Distances _L"=w267:dbl[])
          n71 = Strip Path(path=w274) -> (stripped path=w275:path)  [unwired: 1 out]
          n72 = Format Into String(format string="%s_%s-Report.pdf", w271, w269) -> (resulting string=w270:string)  [unwired: 2 in, 1 out]
          n73 = Array Size(array=w267) -> (size(s)=w268:i32)
          n74 = Build Path(base path=w275, name or relative path=w270) -> (appended path=w273:path)
        }
        frame "Current Page" {
          w282 = u8 1  # One Page
          n75 = Unbundle By Name(w280) -> ("Distance Format"=w279:u8)
          n76 = case shown="1" w279 {
            tunnel: ["%s_%s-Report-%.2fkm.pdf" ("format string") "%s_%s-Report-%.1fmi.pdf" ("format string")] -> w281
            frame 0, Default {
              # "in km"
            }
            frame 1 {
              # "in miles"
            }
          }
          n77 = Strip Path(path=w286) -> (stripped path=w287:path)  [unwired: 1 out]
          n78 = Format Into String(format string=w281, w278, w277, w284) -> (resulting string=w283:string)  [unwired: 2 in, 1 out]
          n79 = Build Path(base path=w287, name or relative path=w283) -> (appended path=w285:path)
        }
      }
      n80 = Unbundle By Name(w166) -> ("Next?"=w231:refnum<vi>, "Previous?"=w230:refnum<vi>, "Run Distance"=w183:refnum<vi>)
      n81 = Unbundle By Name(w166) -> ("Run Distance"=w181:refnum<vi>)
      n82 = Build Array(w231, w230, w183) -> (w229:refnum<vi>[])
      n83 = call <vilib>:"New PDF.vi"("PDF Path"=w196, "Overwrite?"=w205, "Captions"=T13 {"Figure"={"Caption"="Figure", "Separator"="  ", "Position"=enum."Below"}, "Table"={"Caption"="Table", "Separator"="  ", "Position"=enum."Above"}, "Font"={"Name"="", "Size"=-1.0, "Color"=0, "Style"={"Bold"=FALSE, "Italic"=FALSE, "Underline"=FALSE, "Strikeout"=FALSE}, "Type"={"Type&direction"=enum."Select", "Embedded"=FALSE, "Encoding"=""}}}, "Default Font"=T15 {"Name"="Arial", "Size"=12.0, "Color"=0, "Style"={"Bold"=FALSE, "Italic"=FALSE, "Underline"=FALSE, "Strikeout"=FALSE}, "Type"={"Type&direction"=enum."ASCII", "Embedded"=FALSE, "Encoding"=""}}, "At the opening"=T29 {"Page"=0, "Show Bookmarks"=TRUE}, "Default Paragraph"=T20 {" Aligment"=enum."JUSTIFY", "Line spacing"=enum."1.0"}, "error in (no error)"=w165, "Page Setup"=T24 {"Page Size"=1, "Orientation"=enum."Landscape", "Custom Size"={"Width"=216.0, "Height"=279.0}, "Margins"={"Left"=10.0, "Right"=10.0, "Top"=25.0, "Bottom"=25.0}}, "PDF Details"=T23 {"Title"="RailMeasurement RV-HR Report", "Author"="RailMeasurement", "Subject"="", "Keywords"="", "Creator"="RailMeasurement"}, "Permissions"=T12 {"User Password"="", "Owner Password"="", "Printing"=enum."Allow Printing", "Allow Modify Contents"=TRUE, "Allow Copy"=TRUE, "Allow Modify Annotations"=TRUE, "Allow Fill In "=TRUE, "Allow Screen Readers"=TRUE, "Allow Assembly"=TRUE}) -> ("PDF Report"=w197:refnum<class "PDF Report Class.lvclass">, "error out"=w190:errorcluster)  [unwired: 1 in, 3 out]
      n84 = for {
        tunnel: w229 -> [w297] mode=indexing
        shift-right: [w298] -> w180
        shift-left: w190 -> [w299]
        tunnel: [w296] -> w228 mode=indexing
        tunnel: bool[] [FALSE, FALSE, FALSE, TRUE] -> [w295] mode=indexing
        # "Hide Next/Prev Buttons"
        n85 = property class="Ctl"(reference=w297, error in=w299, "Visible"=w295) -> (reference out=w296:refnum<vi>, error out=w298:errorcluster)
      }
      n86 = Bundle("Command"=w226, "Data"=w217) -> (w216:cluster{"Command":string, "Data":variant})  [unwired: 1 in]
      n87 = Obtain Queue(name (unnamed)="Popup Queue", element data type=w216) -> (queue out=w222:refnum<queue>)  [unwired: 3 in, 2 out]
      n88 = case shown="\"Full Report\"" "Command" {
        tunnel: [w242 w247] -> w182
        tunnel: w181 -> [w241 w249]
        tunnel: w180 -> [w240 w248]
        tunnel: [w239 w246] -> w178
        tunnel: [w238 w245] -> w168
        tunnel: w167 -> [w237 _]
        frame "Full Report" {
          # "Initialise back to the start"
          n89 = property class="Slide (strict)"(reference=w241, error in=w240) -> (reference out=w243:refnum<vi>, error out=w244:errorcluster, "Value"=w238:dbl)
          n90 = Unbundle By Name(w237) -> ("Image Distances _L"=w236:dbl[])
          n91 = Array Max & Min(array=w236) -> (min value=w235:dbl)  [unwired: 3 out]
          n92 = property class="Slide (strict)"(reference=w243, error in=w244, "Val(Sgnl)"=w235) -> (reference out=w239:refnum<vi>, error out=w242:errorcluster)
        }
        frame "Current Page" {
          # "Get init position"
          n93 = property class="Slide (strict)"(reference=w249, error in=w248) -> (reference out=w246:refnum<vi>, error out=w247:errorcluster, "Value"=w245:dbl)
        }
      }
      n94 = Open VI Reference(vi path="Main VI Path", error in (no error)=w180) -> (vi reference=w174:refnum<vi>)  [unwired: 4 in, 1 out]
      n95 = case shown="No Error" w182 {
        selector: w182 -> [w251 w252]
        tunnel: [w251 w252] -> w184
        frame No Error {
          n96 = Wait (ms)(milliseconds to wait=u32 2000) -> ()  [unwired: 1 out]
        }
        frame Error {
        }
      }
      n97 = for {
        N: w232 -> [_]
        shift-right: [w334] -> w189
        shift-left: w184 -> [w308]
        shift-right: [w335] -> w194
        shift-left: w197 -> [w333]
        tunnel: w232 -> [w322]
        tunnel: w167 -> [w332]
        shift-right: [w329] -> w191
        shift-left: w222 -> [w331]
        tunnel: [w328] -> w192
        tunnel: "Command" -> [w323]
        tunnel: w174 -> [w311]
        tunnel: [w311] -> w187
        tunnel: w166 -> [w300]
        tunnel: w178 -> [w305]
        tunnel: w175 -> [w303]
        tunnel: "Settings" -> [w302]
        i -> [w304]
        w312 = T32 {"Show?"=TRUE, "Thickness (point)"=0.05, "Color"=13816530}  # Border
        w315 = TRUE  # visible area only?
        # "Create New page for every page > page 1"
        # "Allow UI to update"
        # "Iterate through the pages and append a new page in report / page of data..."
        n98 = Increment(x=w304) -> (x+1=w319:i32)
        n99 = case shown="\"Full Report\"" w323 {
          tunnel: w332 -> [w357 w362]
          tunnel: [w357 w361] -> w307
          tunnel: [w355 w359] -> w321
          tunnel: w322 -> [w355 w359]
          tunnel: w319 -> [_ w360]
          tunnel: [w356 w360] -> w320
          tunnel: w304 -> [_ w358]
          frame "Current Page", Default {
            n100 = Unbundle By Name(w357) -> ("Image"=w356:u16)
          }
          frame "Full Report" {
            n101 = Bundle By Name(cluster=w362, "Image"=w358) -> (w361:T2)
          }
        }
        n102 = case shown="0" w304 {
          tunnel: [w336 w348] -> w310
          tunnel: [w339 w347] -> w309
          tunnel: w308 -> [w340 w346]
          tunnel: w300 -> [_ w345]
          tunnel: w307 -> [w337 w342]
          tunnel: [w337 w344] -> w306
          tunnel: w305 -> [w338 _]
          tunnel: w303 -> [_ _]
          tunnel: w302 -> [_ w341]
          frame 0 {
            n103 = property class="Slide (strict)"(reference=w338, error in=w340) -> (error out=w339:errorcluster, "Value"=w336:dbl)  [unwired: 1 out]
          }
          frame 1, Default {
            n104 = call "RVHR - New Distance.vi"("Command"=enum16{"Next", "Previous"}."Next", "Local Data in"=w342, "UI Refs"=w345, "error in (no error)"=w346, "Supervisory Config Cluster In"=w341) -> ("error out"=w347:errorcluster, "New Distance"=w348:dbl, "Local Data out"=w344:T2)  [unwired: 4 in]
          }
        }
        n105 = call "RVHR - Get Current Images.vi"("Local Data in"=w306, "UI Refs"=w300, "error in (no error)"=w309, 11:w310) -> ("error out"=w301:errorcluster)  [unwired: 6 in, 1 out]
        n106 = Divide(x=w320, y=w321) -> (x/y=w326:dbl)
        n107 = case shown="No Error" w301 {
          selector: w301 -> [w364 w365]
          tunnel: [w364 w365] -> w330
          frame No Error {
            n108 = Wait (ms)(milliseconds to wait=u32 100) -> ()  [unwired: 1 out]
          }
          frame Error {
          }
        }
        n109 = Multiply(x=w326, y=100.0) -> (x*y=w324:dbl)
        n110 = Bundle By Name(cluster=cluster{"Command":string, "Data":variant} {"Command"="Update Progress", "Data"=variant} ("output cluster"), "Data"=w324) -> (w327:cluster{"Command":string, "Data":variant})
        n111 = case shown="1, Default" w304 {
          tunnel: w333 -> [w350 w351]
          tunnel: [w350 w352] -> w317
          tunnel: [w349 w353] -> w316
          tunnel: w330 -> [w349 w354]
          frame 0 {
          }
          frame 1, Default {
            n112 = call <vilib>:"Append New Page.vi"("PDF Report"=w351, "error in (no error)"=w354) -> ("PDF Report duplicate"=w352:refnum<class "PDF Report Class.lvclass">, "error OUT"=w353:errorcluster)  [unwired: 12 out]
          }
        }
        n113 = Enqueue Element(queue=w331, element=w327, error in (no error)=w330) -> (queue out=w329:refnum<queue>, error out=w328:errorcluster)  [unwired: 1 in, 1 out]
        n114 = call <vilib>:"Append Front Panel Image.vi"("PDF Report IN"=w317, "Scale (%)"=sgl 100.0, "Border"=w312, "VI reference"=w311, "visible area only? (T)"=w315, "error in (no error)"=w316, "Position and indentation"=T30 {"Alignment"=enum."Center", "X "=0.0, "Y"=0.0, "Indentation"=0.0}) -> ("PDF Report OUT"=w335:refnum<class "PDF Report Class.lvclass">, "error out"=w334:errorcluster)  [unwired: 7 in]
      }
      n115 = Bundle By Name(cluster=cluster{"Command":string, "Data":variant} {"Command"="Update Progress", "Data"=variant} ("output cluster"), "Data"=u8 0 ("Progress")) -> (w223:cluster{"Command":string, "Data":variant})
      n116 = Enqueue Element(queue=w222, element=w223, error in (no error)=w180) -> (queue out=w215:refnum<queue>, error out=w221:errorcluster)  [unwired: 1 in, 1 out]
      n117 = call "Print Popup.vi"("error in"=w221, "queue in"=w215) -> ("error out"=w225:errorcluster, "queue out"=w224:refnum<queue>)  [unwired: 8 in]
      n118 = Close Reference(reference=w187, error in (no error)=w189) -> (error out=w188:errorcluster)
      n119 = Release Queue(queue=w224, error in (no error)=w225) -> ()  [unwired: 1 in, 3 out]
      n120 = for {
        N: 3 -> [_]
        tunnel: w228 -> [w292] mode=indexing
        shift-right: [w293] -> w195
        shift-left: w188 -> [w294]
        tunnel: [w290] -> _ mode=indexing
        # "Show Next/Prev Buttons"
        n121 = property class="Ctl"(reference=w292, error in=w294, "Visible"=TRUE) -> (reference out=w290:refnum<vi>, error out=w293:errorcluster)
      }
      n122 = call <vilib>:"Close PDF.vi"("PDF Report"=w194, "error in (no error)"=w195) -> ("Path"=w193:path, "error out"=w171:errorcluster)  [unwired: 12 out]
      n123 = call "RVHR - Get Current Images.vi"("Local Data in"=w167, "UI Refs"=w166, "error in (no error)"=w171, 11:w168) -> ("error out"=w170:errorcluster)  [unwired: 6 in, 1 out]
      n124 = Unbundle By Name(w166) -> ("Run Distance"=w169:refnum<vi>)
      n125 = property class="Slide (strict)"(reference=w169, error in=w170, "Value"=w168) -> ()  [unwired: 2 out]
      n126 = Path To String(path=w193) -> (string=w207:string)
      n127 = Bundle By Name(cluster=cluster{"Command":string, "Data":variant} {"Command"="Filename", "Data"=variant} ("output cluster"), "Data"=w207) -> (w208:cluster{"Command":string, "Data":variant})
      n128 = Enqueue Element(queue=w191, element=w208, error in (no error)=w192) -> (queue out=w211:refnum<queue>, error out=w213:errorcluster)  [unwired: 1 in, 1 out]
      n129 = case shown="Error" w213 {
        selector: w213 -> [w263 w266]
        tunnel: [w264 w265] -> w212
        tunnel: w211 -> [w264 w265]
        tunnel: [w263 w266] -> w210
        frame No Error {
          n130 = Wait (ms)(milliseconds to wait=u32 4000) -> ()  [unwired: 1 out]
        }
        frame Error {
        }
      }
      n131 = Enqueue Element(queue=w212, element=cluster{"Command":string, "Data":variant} {"Command"="Exit", "Data"=variant} ("output cluster"), error in (no error)=w210) -> ()  [unwired: 1 in, 3 out]
    }
    frame Enabled {
    }
  }
  n132 = call "RVHR_Export Results_ExaPromPDF.vi"("Local Data"=w1, "appended path"=w5, "error in (no error)"=w20, "Feature Table"=w21) -> ("error out"=w4:errorcluster)  [unwired: 7 in]
  "error out" <- w4
  n133 = Bundle("Command"=w17, "Data"=w18) -> (w19:cluster{"Command":string, "Data":variant})  [unwired: 1 in]
  n134 = Obtain Queue(name (unnamed)="Popup Queue", element data type=w19, error in (no error)=w4) -> (queue out=w9:refnum<queue>, error out=w8:errorcluster)  [unwired: 2 in, 1 out]
  n135 = call "Print Popup.vi"("error in"=w8, "queue in"=w9) -> ()  [unwired: 8 in, 2 out]
  n136 = Path To String(path=w5) -> (string=w15:string)
  n137 = Bundle By Name(cluster=cluster{"Command":string, "Data":variant} {"Command"="Filename", "Data"=variant} ("output cluster"), "Data"=w15) -> (w14:cluster{"Command":string, "Data":variant})
  n138 = Enqueue Element(queue=w9, element=w14, error in (no error)=w8) -> (queue out=w7:refnum<queue>, error out=w6:errorcluster)  [unwired: 1 in, 1 out]
  n139 = case shown="Error" w6 {
    selector: w6 -> [w367 w370]
    tunnel: [w368 w369] -> w11
    tunnel: w7 -> [w368 w369]
    tunnel: [w367 w370] -> w12
    frame No Error {
      n140 = Wait (ms)(milliseconds to wait=u32 4000) -> ()  [unwired: 1 out]
    }
    frame Error {
    }
  }
  n141 = Enqueue Element(queue=w11, element=cluster{"Command":string, "Data":variant} {"Command"="Exit", "Data"=variant} ("output cluster"), error in (no error)=w12) -> (error out=w2:errorcluster)  [unwired: 1 in, 2 out]
  n142 = case shown="No Error" w2 {
    selector: w2 -> [w371 w373]
    tunnel: [w371 w373] -> _
    frame No Error {
      # "Deallocate Memory"
      n143 = Request Deallocation(TRUE ("flag")) -> ()
    }
    frame Error {
    }
  }
